vi "UpdateNextTestFileForHBM.vi"(4 "entrée d'erreur":errorcluster, 6 "NextTestNum":u32, 7 "NomProjet":string) -> (0 "sortie d'erreur":errorcluster)   [LabVIEW 2017]
uses:
  DefDeType/WhichPath.ctl
panel:
  out "cheminProchainFichier":path
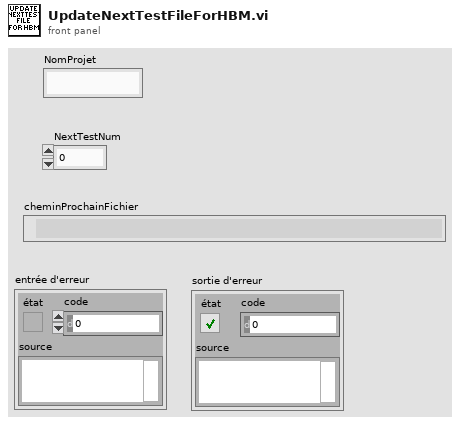
[diagram p1: front panel]
types:
  T1 = enum16{"open", "replace", "create", "open or create", "replace or create", "replace or create with confirmation"}
  T2 = typedef "WhichPath.ctl" = enum16{"DossierProjet", "Config", "Meas", "MeasPCI", "MeasCRIO1", "MeasCRIO2", "MeasQualisys", "MeasHBM", "MeasTDMS", "Fig", "Res"}
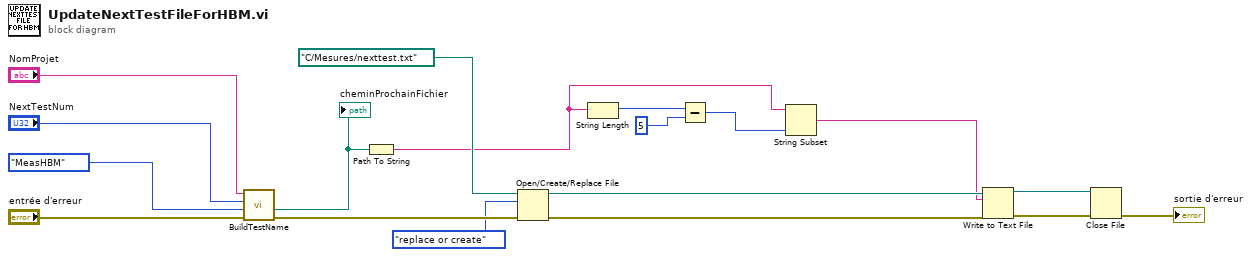
[diagram p0: block diagram]
diagram:
  n1 = call "BuildTestName.vi"("entrée d'erreur"="entrée d'erreur", "WhichPath?"=WhichPath."MeasHBM", "NextTestNum"="NextTestNum", "NomProjet"="NomProjet") -> ("sortie d'erreur"=w14:errorcluster, "cheminProchainFichier"=w8:path)  [unwired: 1 in, 2 out]
  "cheminProchainFichier" <- w8
  n2 = Path To String(path=w8) -> (string=w1:string)
  n3 = Open/Create/Replace File(file path (use dialog)=path "C:/Mesures/nexttest.txt" ("chemin du fichier (utiliser une boîte de dialogue)"), error in=w14, operation (0:open)=T1."replace or create" ("opération (0 : open)")) -> (refnum out=w10:refnum<file>, error out=w13:errorcluster)  [unwired: 3 in, 1 out]
  n4 = String Length(string=w1) -> (length=w5:i32)
  n5 = Subtract(x=w5, y=5) -> (x-y=w3:i32)
  n6 = String Subset(string=w1, length (rest)=w3) -> (substring=w2:string)  [unwired: 1 in]
  n7 = Write to Text File(file (use dialog)=w10, text=w2, error in=w13) -> (refnum out=w7:refnum<file>, error out=w12:errorcluster)  [unwired: 1 in, 1 out]
  n8 = Close File(refnum=w7, error in=w12) -> (error out=→"sortie d'erreur":errorcluster)  [unwired: 1 out]
